vi "52-lfs-r1_begin.vi"(8 "error in (no error)":errorcluster, 9 "Position in":T1) -> (0 "error out":errorcluster, 1 "Position out":T1, 4 "side?":bool)   [LabVIEW 2019]
uses:
  subVI/move/position cluster.ctl
  subVI/move control/move and align/move_cluster.ctl
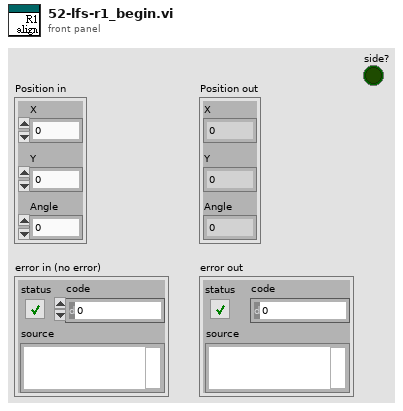
[diagram p1: front panel]
types:
  T1 = typedef "position cluster.ctl" = cluster{"X":dbl, "Y":dbl, "Angle":dbl}
  T2 = typedef "move_cluster.ctl" = cluster{"X":dbl, "Y":dbl, "degree":dbl, "speed":dbl}
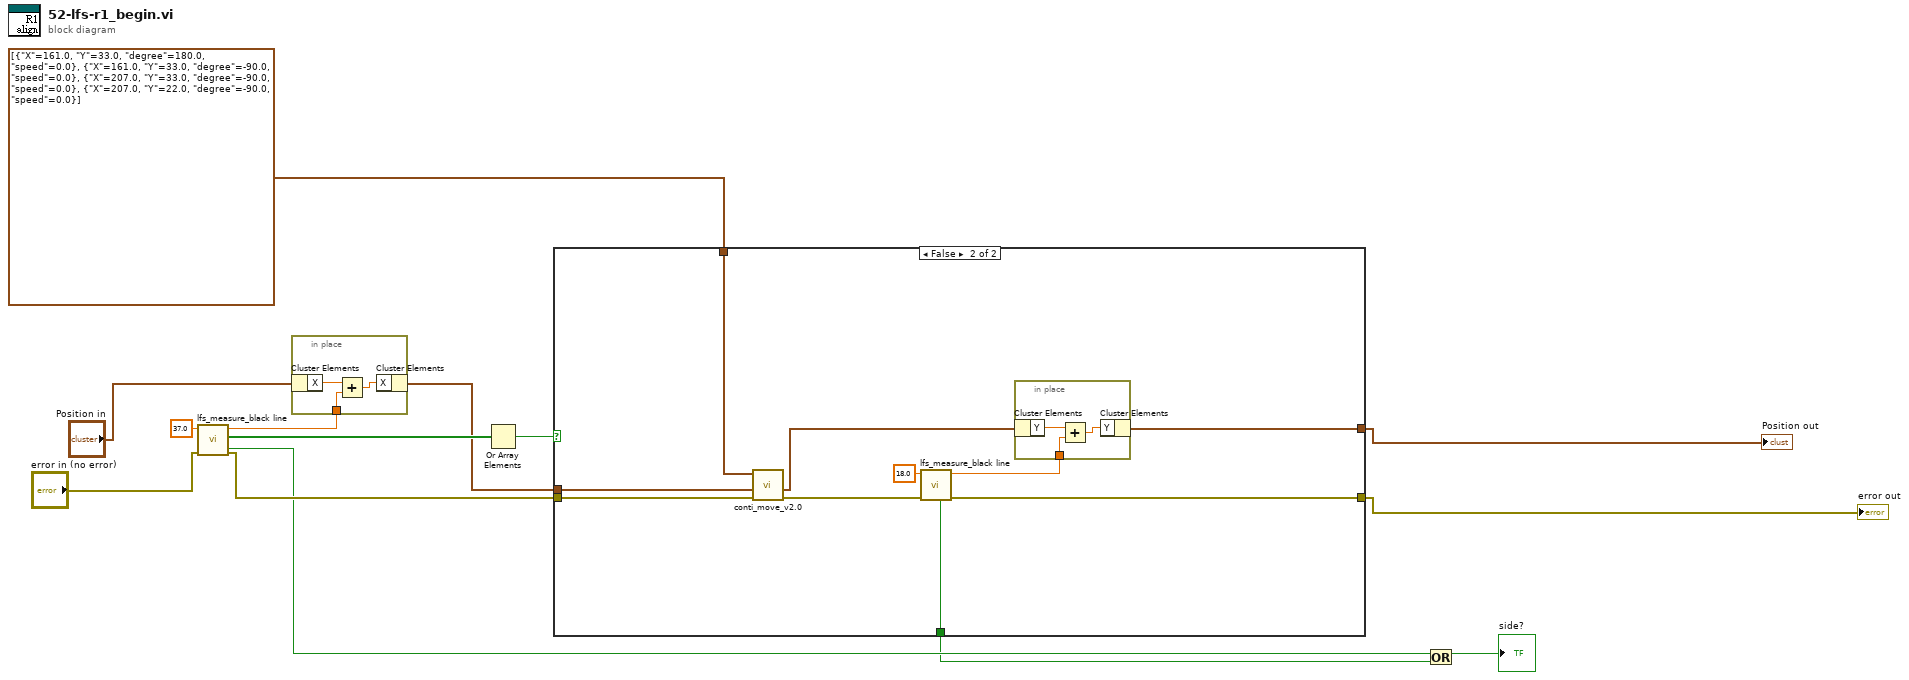
[diagram p0: block diagram]
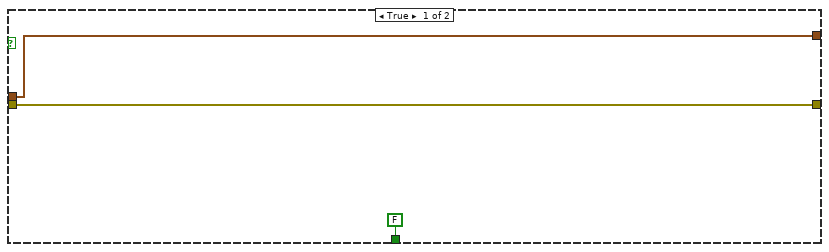
[diagram p2: hidden frame]
diagram:
  n1 = call "lfs_measure_black line.vi"("error in (no error)"="error in (no error)", "limit"=37.0) -> ("error out"=w7:errorcluster, "0:R 1:L"=w9:bool[], "move cm"=w14:dbl, "side?"=w4:bool)  [unwired: 6 in]
  n2 = in-place {
    in-place-border: w14 -> [w16]
    n3 = in-place-cluster #1("Position in") -> ("X"=w17:dbl)
    n4 = Add(x=w17, y=w16) -> (x+y=w15:dbl)
    n5 = in-place-cluster #1("X"=w15) -> (w8:T1)
  }
  n6 = Or Array Elements(Boolean array=w9) -> (logical OR=w1:bool)
  n7 = case shown="False" w1 {
    tunnel: T2[] [{"X"=161.0, "Y"=33.0, "degree"=180.0, "speed"=0.0}, {"X"=161.0, "Y"=33.0, "degree"=-90.0, "speed"=0.0}, {"X"=207.0, "Y"=33.0, "degree"=-90.0, "speed"=0.0}, {"X"=207.0, "Y"=22.0, "degree"=-90.0, "speed"=0.0}] ("route") -> [_ w30]
    tunnel: w8 -> [w19 w29]
    tunnel: w7 -> [w20 w28]
    tunnel: [w20 w23] -> w5
    tunnel: [w19 w22] -> w6
    tunnel: [FALSE ("side?") w21] -> w2
    frame True {
    }
    frame False {
      n8 = call "conti_move_v2.0.vi"("error in (no error)"=w28, "Position"=w29, "route"=w30) -> ("error out"=w24:errorcluster, "Position out"=w25:T1)  [unwired: 7 in]
      n9 = call "lfs_measure_black line.vi"("error in (no error)"=w24, "limit"=18.0) -> ("error out"=w23:errorcluster, "move cm"=w26:dbl, "side?"=w21:bool)  [unwired: 6 in, 1 out]
      n10 = in-place {
        in-place-border: w26 -> [w32]
        n11 = in-place-cluster #2(w25) -> ("Y"=w33:dbl)
        n12 = Add(x=w33, y=w32) -> (x+y=w31:dbl)
        n13 = in-place-cluster #2("Y"=w31) -> (w22:T1)
      }
    }
  }
  "Position out" <- w6
  "error out" <- w5
  n14 = Or(x=w4, y=w2) -> (x .or. y?=→"side?":bool)
